vi "Do Something.vi"(8 "error in (no error)":errorcluster, 11 "ByRef Mul in":refnum<class "ByRef Mul.lvclass">) -> (0 "error out":errorcluster, 3 "ByRef Mul out":refnum<class "ByRef Mul.lvclass">)   [LabVIEW 2012, in "ByRef Mul.lvclass"]
uses:
  ByRef Mul.lvclass
  ByRef Base/ByRef Base.lvclass
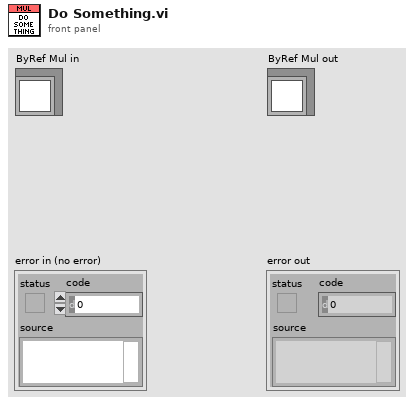
[diagram p1: front panel]
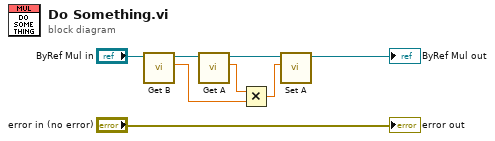
[diagram p0: block diagram]
diagram:
  n1 = call "Get B.vi"("ByRef Base in"="ByRef Mul in") -> ("B"=w1:dbl, "ByRef Base out"=w2:refnum<class "ByRef Mul.lvclass">)  [unwired: 8 in, 1 out]
  n2 = call "Get A.vi"("ByRef Base in"=w2) -> ("Numeric"=w5:dbl, "ByRef Base out"=w8:refnum<class "ByRef Mul.lvclass">)  [unwired: 8 in, 1 out]
  n3 = Multiply(x=w5, y=w1) -> (x*y=w4:dbl)
  n4 = call "Set A.vi"("Numeric"=w4, "ByRef Base in"=w8) -> ("ByRef Base out"=→"ByRef Mul out":refnum<class "ByRef Mul.lvclass">)  [unwired: 8 in, 1 out]
  "error out" <- "error in (no error)"
